vi "3D-BasePointMessage.vi"(10 "Base Poit 2":cluster{"X":dbl, "Y":dbl, "Z":dbl}[](array[cluster]), 11 "Base Poit":cluster{"X":dbl, "Y":dbl, "Z":dbl}[](array[cluster])) -> (3 "添加的数组":string[](array[string]))   [LabVIEW 2015]
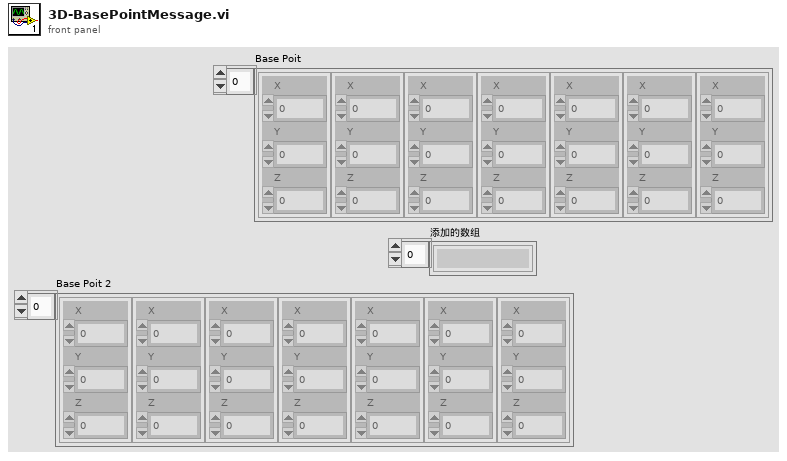
[diagram p1: front panel]
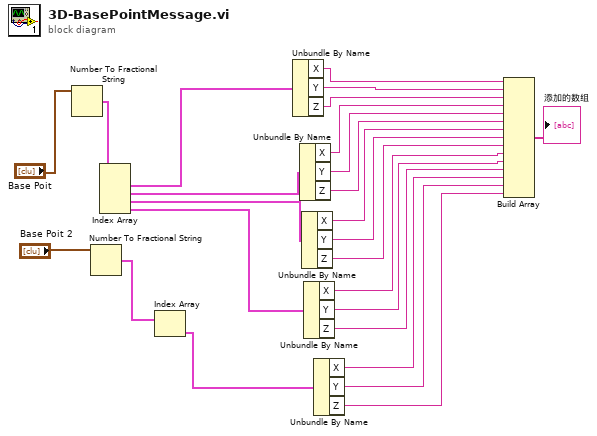
[diagram p0: block diagram]
diagram:
  n1 = Number To Fractional String(number="Base Poit") -> (F-format string=w23:cluster{"X":string, "Y":string, "Z":string}[])  [unwired: 3 in]
  n2 = Number To Fractional String(number="Base Poit 2") -> (F-format string=w5:cluster{"X":string, "Y":string, "Z":string}[])  [unwired: 3 in]
  n3 = Index Array(array=w23) -> (element #1=w25:cluster{"X":string, "Y":string, "Z":string}, element #2=w22:cluster{"X":string, "Y":string, "Z":string}, element #3=w21:cluster{"X":string, "Y":string, "Z":string}, element #4=w20:cluster{"X":string, "Y":string, "Z":string})  [unwired: 4 in]
  n4 = Index Array(array=w5) -> (element=w4:cluster{"X":string, "Y":string, "Z":string})  [unwired: 1 in]
  n5 = Unbundle By Name(w25) -> ("X"=w19:string, "Y"=w18:string, "Z"=w17:string)
  n6 = Unbundle By Name(w22) -> ("X"=w16:string, "Y"=w15:string, "Z"=w14:string)
  n7 = Unbundle By Name(w21) -> ("X"=w13:string, "Y"=w12:string, "Z"=w11:string)
  n8 = Unbundle By Name(w20) -> ("X"=w10:string, "Y"=w9:string, "Z"=w8:string)
  n9 = Unbundle By Name(w4) -> ("X"=w3:string, "Y"=w2:string, "Z"=w1:string)
  n10 = Build Array(w19, w18, w17, w16, w15, w14, w13, w12, w11, w10, w9, w8, w3, w2, w1) -> (→"添加的数组":string[])
